vi "Concacenate String Array.vi"(4 "Max Number of Elements (None: -1)":i32=-1, 6 "Separator (TAB)":string="\t", 8 "Suffix (\"\")":string, 10 "String Array":string[](array[string]), 11 "Prefix (\"\")":string) -> (2 "Formatted String":string)   [LabVIEW 2019]
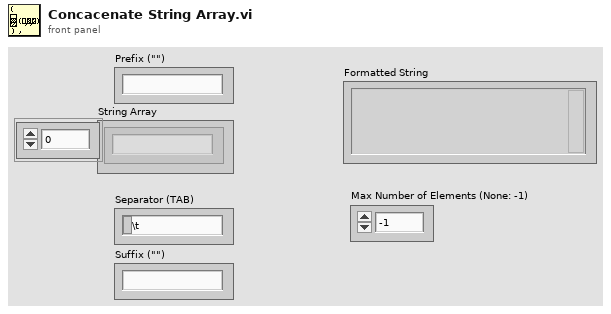
[diagram p1: front panel]
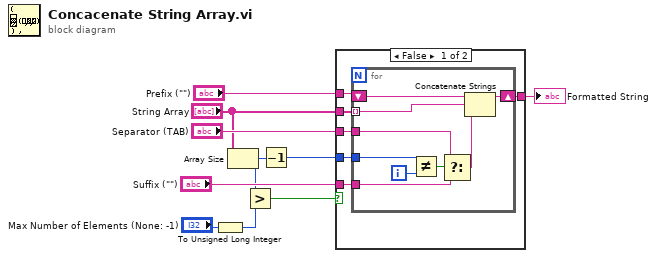
[diagram p0: block diagram]
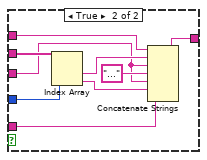
[diagram p2: hidden frame]
diagram:
  n1 = To Unsigned Long Integer(number="Max Number of Elements (None: -1)") -> (unsigned 32bit integer=w2:u32)
  n2 = Array Size(array="String Array") -> (size(s)=w4:i32)
  n3 = Greater?(x=w4, y=w2) -> (0:w1:bool)
  n4 = Decrement(x=w4) -> (x-1=w6:i32)
  n5 = case shown="False" w1 {
    tunnel: [w16 w26] -> w10
    tunnel: "Prefix (\"\")" -> [w15 w32]
    tunnel: "Separator (TAB)" -> [w14 w28]
    tunnel: "String Array" -> [w13 w34]
    tunnel: w6 -> [w12 w33]
    tunnel: "Suffix (\"\")" -> [w11 w27]
    frame False {
      n6 = for {
        tunnel: w13 -> [w24] mode=indexing
        shift-right: [w23] -> w16
        shift-left: w15 -> [w25]
        tunnel: w14 -> [w18]
        tunnel: w12 -> [w22]
        tunnel: w11 -> [w19]
        i -> [w21]
        n7 = Not Equal?(x=w22, y=w21) -> (x != y?=w20:bool)
        n8 = Select(t=w18, s=w20, f=w19) -> (s? t:f=w17:string)
        n9 = Concatenate Strings(w25, w24, w17) -> (w23:string)
      }
    }
    frame True {
      n10 = Index Array(array=w34, index #2=w33) -> (element #1=w31:string, element #2=w29:string)  [unwired: 1 in]
      n11 = Concatenate Strings(w32, w31, w28, "..." ("string"), w28, w29, w27) -> (w26:string)
    }
  }
  "Formatted String" <- w10
